vi "Apollo 3 v1.vi"() -> ()   [LabVIEW 2014]
uses:
  Global_vars.vi
panel:
  out "Test":dbl
  out "RL Command":dbl
  out "FR Command":dbl
  in  "Reorder Sim":i16=132
  out "Sim Lats and Longs":dbl[][](array[numeric]) format="%#_8g"
  in  "?":bool
  in  "Trail on/off":bool=TRUE
  in  "sim path":path=path "C:/Users/robotics/Desktop/Apollo II IGVC 2016 code/APOLLO 3 with fixed directory structure/Sim Drawings/IGVC II Test Paint.bmp"
  in  "Real WP Lats and Longs":dbl[][](array[numeric])=[[37.2651198, 81.2424197], [37.2652566, 81.2421218], [37.2653258, 81.2419709], [37.265326, 81.241971], [37.265326, 81.241971], [37.265326, 81.241971], [37.265326, 81.241971], [37.265326, 81.241971], [37.265326, 81.241971], [37.265326, 81.241971]] format="%#_8g"
  out "?":bool[](array[boolean])
  out "Robot Information":dbl[](array[numeric]) format="%#_8g"
  in  "Parameters":dbl[](array[numeric])=[2.0, 100.0, 10.0, 100.0, 30.0, 100.0, 3.0, 270.0, 37.1526, 81.2675, 7.3, 0.0, 60.0, 40.0, 0.0, 0.0, 0.0, 0.0, 0.0, 0.0]
  in  "GPS Port":refnum<visa-resource-name>="COM14"
  in  "Compass Port":refnum<visa-resource-name>="COM11"
  in  "Tx Prop  Port":refnum<visa-resource-name>="COM4"
  in  "Extra Port":refnum<visa-resource-name>="COM12"
  in  "Hokuyo Port":refnum<visa-resource-name>="COM13"
  out "main loop time":dbl=0.026001453399658203
  in  "Use ?\nOff       On":bool[](array[boolean])=[TRUE, TRUE, TRUE, TRUE, TRUE, FALSE]
  out "Local Map":picture
  in  "Num of WPs":i16=10
  out "Global Map":picture
  in  "START":bool
  in  "Mode:":bool
  out "WP Map":cluster{"WP Longs":dbl[], "WP Lats":dbl[]}(graph)
  out "loop iteration":i64=9025
  in  "STOP":bool
  # "Apollo 3 v1"
  # "Constants"
  # "Fat(0)"
  # "Setup"
  # "WT: Ahead(1)"
  # "WT: Gap(2)"
  # "WT: Slant(3)"
  # "GPS"
  # "WT: Dist(4)"
  # "LMS"
  # "WT: WP(5)"
  # "Vision"
  # "Sim Vel(6)"
  # "Tx Prop"
  # "Sim Hdg0(7)"
  # "Sim Lat0(8)"
  # "Comp"
  # "Sim Long0(9)"
  # "Extra"
  # "Sim Dev0(10)"
  # "Ang Bias(11)"
  # "Vel Bias(12)"
  # "Sim"
  # "Real"
  # "Run Time Robot Data"
  # "Goal x(13)"
  # "Goal y (14)"
  # "Robot Lat"
  # "Objx (15)"
  # "Robot Long"
  # "Objy (16)"
  # "Robot Heading"
  # "Old GPS L (17)"
  # "Robot Path Angle"
  # "Old GPS l (18)"
  # "Robot Speed"
  # "Simulation Settings"
  # "Old Heading (19)"
  # "Data Sent to Propeller"
  # "Angle to WP"
  # "Robot Trail:"
  # "Dist in Meters to WP"
  # "Pause"
  # "WP Number"
  # "Path to simulation BMP:"
  # "Next WP Lat"
  # "Resume"
  # "Next WP Long"
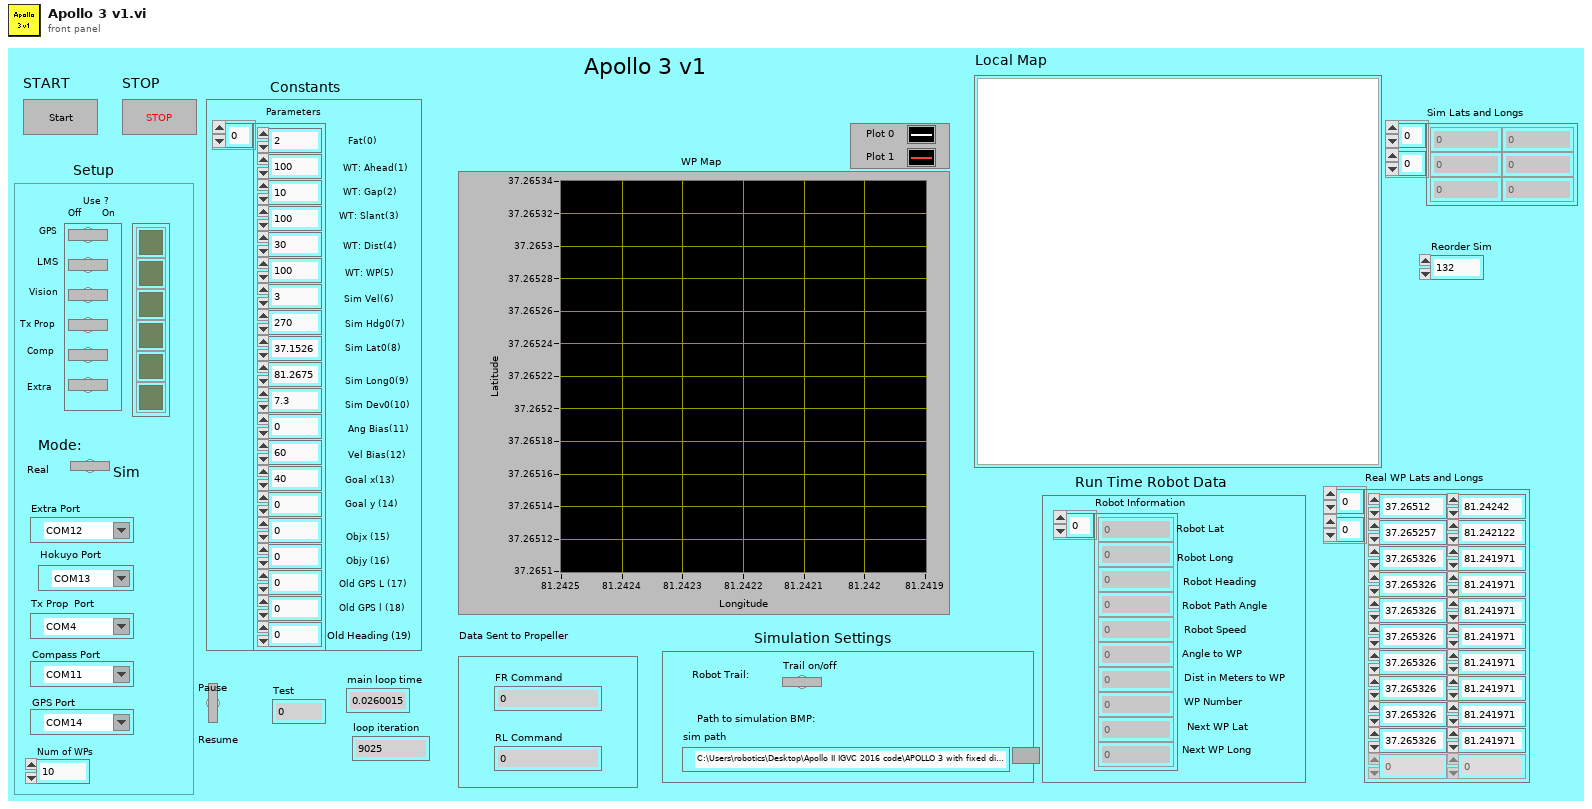
[diagram p1: front panel]
types:
  T1 = cluster{"     Use ?\nOff       On":bool[], "Mode:":bool, "Extra Port":refnum<visa-resource-name>, "Hokuyo Port":refnum<visa-resource-name>, "Tx Prop  Port":refnum<visa-resource-name>, "Compass Port":refnum<visa-resource-name>, "GPS Port":refnum<visa-resource-name>}
  T2 = cluster{"     Use ?\nOff       On":bool[], "Mode:":bool, "Extra Port":refnum<visa-resource-name>, "Hokuyo Port":refnum<visa-resource-name>, "Tx Prop  Port":refnum<visa-resource-name>, "Compass Port":refnum<visa-resource-name>, "GPS Port":refnum<visa-resource-name>, "Num of WPs":i16, "WP Lats and Longs":cluster{"WP Lats":dbl[], "WP Longs":dbl[]}, "Obst Lats and Longs":cluster{"Obst Lats":dbl[], "Obst Longs":dbl[]}, "Parameters":dbl[], "GPS Data":dbl[], "Compass":dbl, "LMS Vector":dbl[], "Vision Vector":dbl[], "Direction Cmd":dbl, "Speed Cmd":dbl, "WP Vector":dbl[], "WP Number":i32, "Extra":i16, "SW Map":i32[][], "Path Cluster":cluster{"Path x node":dbl[], "Path y node":dbl[]}, "Sim Course":i8[][]}
  T3 = cluster{"     Use ?\nOff       On":bool[], "Mode:":bool, "Extra Port":refnum<visa-resource-name>, "Hokuyo Port":refnum<visa-resource-name>, "Tx Prop Port":refnum<visa-resource-name>, "Compass Port":refnum<visa-resource-name>, "GPS Port":refnum<visa-resource-name>, "Num of WPs":i16, "WP Lats and Longs":cluster{"WP Lats":dbl[], "WP Longs":dbl[]}, "Obst Lats and Longs":cluster{"Obst Lats":dbl[], "Obst Longs":dbl[]}, "Parameters":dbl[], "GPS Data":dbl[], "Compass":dbl, "LMS Vector":dbl[], "Vision Vector":dbl[], "Direction Cmd":dbl, "Speed Cmd":dbl, "WP Vector":dbl[], "WP Number":i32, "Extra":i16, "SW Map":i32[][], "Path Cluster":cluster{"Path x node":dbl[], "Path y node":dbl[]}, "Sim Course":i8[][]}
  T4 = cluster{"     Use ?\nOff       On":bool[], "Mode:":bool, "Extra Port":refnum<visa-resource-name>, "Hokuyo Port":refnum<visa-resource-name>, "Prop  Port":refnum<visa-resource-name>, "Compass Port":refnum<visa-resource-name>, "GPS Port":refnum<visa-resource-name>, "Num of WPs":i16, "WP Lats and Longs":cluster{"WP Lats":dbl[], "WP Longs":dbl[]}, "Obst Lats and Longs":cluster{"Obst Lats":dbl[], "Obst Longs":dbl[]}, "Parameters":dbl[], "GPS Data":dbl[], "Compass":dbl, "LMS Vector":dbl[], "Vision Vector":dbl[], "Direction Cmd":dbl, "Speed Cmd":dbl, "WP Vector":dbl[], "WP Number":i32, "Extra":i16, "SW Map":i32[][], "Path Cluster":cluster{"Path x node":dbl[], "Path y node":dbl[]}, "Sim Course":i8[][]}
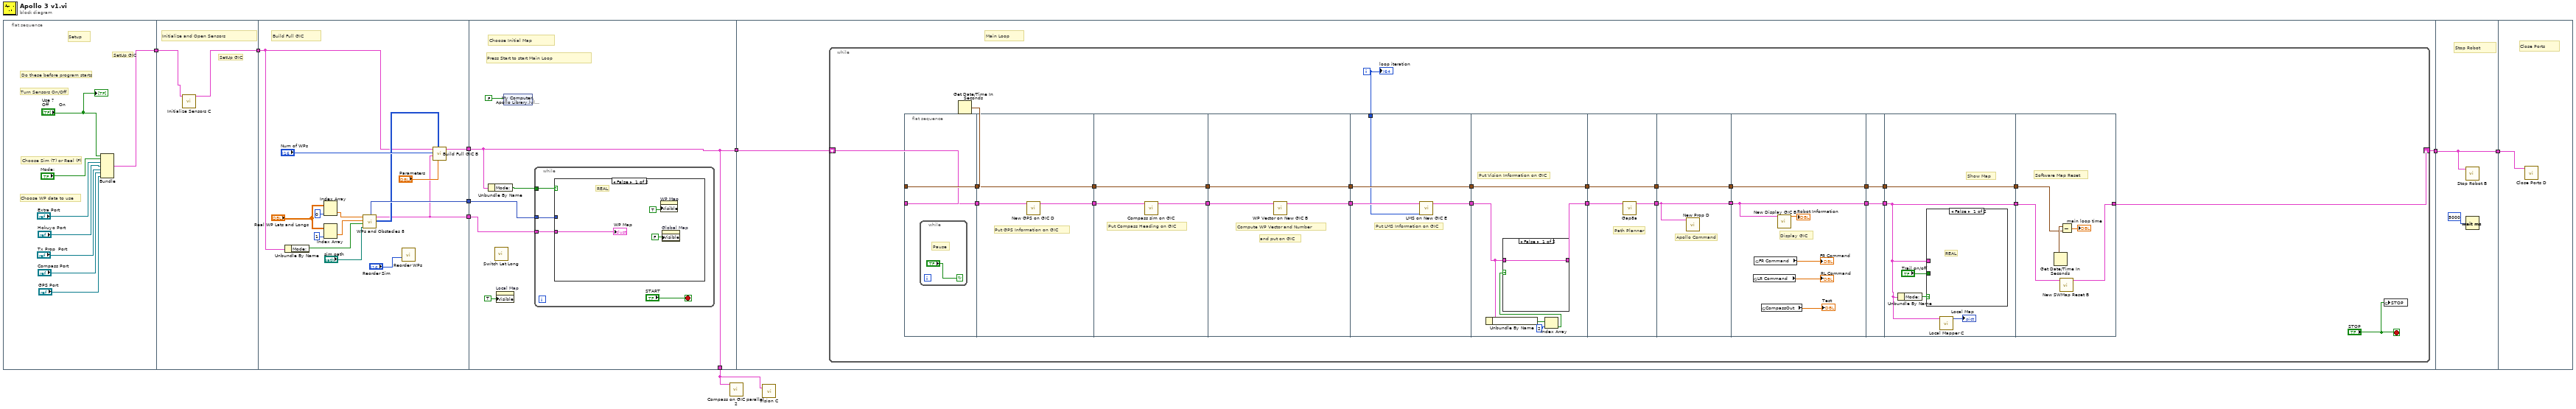
[diagram p0: block diagram]
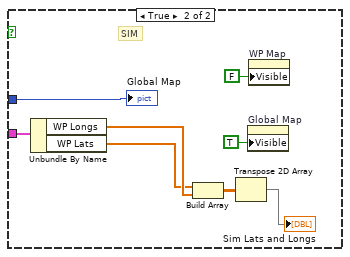
[diagram p2: hidden frame]
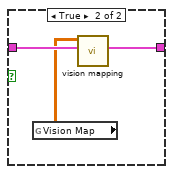
[diagram p3: hidden frame]
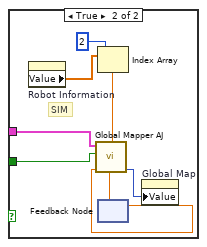
[diagram p4: hidden frame]
diagram:
  n1 = flat-sequence {
    tunnel: [w12] -> w9
    tunnel: w9 -> [w19]
    tunnel: [w18] -> w5
    tunnel: w5 -> [w24]
    tunnel: [w34] -> w4
    tunnel: [w32] -> w3
    tunnel: [w20] -> w2
    tunnel: [w35] -> w8
    tunnel: w2 -> [w36]
    tunnel: w3 -> [w38]
    tunnel: w4 -> [w35]
    tunnel: [w35] -> w1
    tunnel: [w57] -> w7
    tunnel: w8 -> [w56]
    tunnel: w7 -> [w143]
    tunnel: [w143] -> w6
    tunnel: w6 -> [w144]
    frame #0 {
      # "SetUp GIC"
      # "Choose WP data to use"
      # "Do these before program starts"
      # "Choose Sim (T) or Real (F)"
      # "Turn Sensors On/Off"
      # "Setup"
      n2 = Bundle("Use ?\nOff       On"="Use ?\nOff       On", "Mode:"="Mode:", "Extra Port"="Extra Port", "Hokuyo Port"="Hokuyo Port", "Tx Prop  Port"="Tx Prop  Port", "Compass Port"="Compass Port", "GPS Port"="GPS Port") -> (w12:T1)  [unwired: 1 in]
      "?" <- "Use ?\nOff       On"
    }
    frame #1 {
      # "SetUp GIC"
      # "Initialize and Open Sensors"
      n3 = call "Initialize Sensors C.vi"(11:w19) -> (3:w18:T1)  [unwired: 10 in]
    }
    frame #2 {
      # "Build Full GIC"
      n4 = Unbundle By Name(w24) -> ("Mode:"=w23:bool)
      n5 = Index Array(array="Real WP Lats and Longs", index (col)=1 ("disabled index (col)")) -> (element=w26:dbl[])  [unwired: 1 in]
      n6 = Index Array(array="Real WP Lats and Longs", index (col)=0 ("disabled index (col)")) -> (element=w27:dbl[])  [unwired: 1 in]
      n7 = call "WPs and Obstacles 8.vi"("sim path"="sim path", "Mode"=w23, "WP Real Longs"=w26, "WP Real Lats"=w27) -> ("Sim Matrx"=w31:u8[][], "WP Map"=w20:cluster{"WP Longs":dbl[], "WP Lats":dbl[]}, "Sim Course"=w32:picture)  [unwired: 3 in, 1 out]
      n8 = call "Reorder WPs.vi"("ReOrder Sim 123"="Reorder Sim") -> ()  [unwired: 10 in, 1 out]
      n9 = call "Build Full GIC B.vi"("Parameters"="Parameters", "Sim Course"=w31, "WP Lats and Longs"=w20, "Num of WPs"="Num of WPs", 11:w24) -> ("Full GIC"=w34:T2)  [unwired: 6 in]
    }
    frame #3 {
      # "Choose Initial Map"
      # "Press Start to start Main Loop"
      n10 = Unbundle By Name(w35) -> ("Mode:"=w37:bool)
      n11 = call "Switch Lat Long.vi"() -> ()  [unwired: 1 in, 1 out]
      n12 = property on="Local Map" class="Pict"("Visible"=TRUE) -> ()  [unwired: 2 in, 2 out]
      n13 = shared-variable "My Computer\\Apollo Library.lvlib\\stop"(FALSE) -> ()  [unwired: 1 in, 1 out]
      n14 = while {
        tunnel: w38 -> [w42]
        tunnel: w36 -> [w41]
        tunnel: w37 -> [w43]
        stop <- "START" stop-if-true
        n15 = case shown="False" w43 {
          tunnel: w42 -> [_ w55]
          tunnel: w41 -> [w47 w52]
          frame False {
            # "REAL"
            n16 = property on="WP Map" class="XYGraph (strict)"("Visible"=TRUE) -> ()  [unwired: 2 in, 2 out]
            n17 = property on="Global Map" class="Pict"("Visible"=FALSE) -> ()  [unwired: 2 in, 2 out]
            "WP Map" <- w47
          }
          frame True {
            # "SIM"
            n18 = Unbundle By Name(w52) -> ("WP Longs"=w51:dbl[], "WP Lats"=w50:dbl[])
            n19 = Build Array(w50, w51) -> (w49:dbl[][])
            n20 = Transpose 2D Array(2D array=w49) -> (transposed array=→"Sim Lats and Longs":dbl[][])
            n21 = property on="Global Map" class="Pict"("Visible"=TRUE) -> ()  [unwired: 2 in, 2 out]
            n22 = property on="WP Map" class="XYGraph (strict)"("Visible"=FALSE) -> ()  [unwired: 2 in, 2 out]
            "Global Map" <- w55
          }
        }
      }
    }
    frame #4 {
      # "Main Loop"
      n23 = while {
        shift-right: [w67] -> w57
        shift-left: w56 -> [w75]
        i -> [w66]
        stop <- "STOP" stop-if-true
        n24 = flat-sequence {
          tunnel: w75 -> [w85]
          tunnel: w78 -> [w86]
          tunnel: [w86] -> w61
          tunnel: [w85] -> w60
          tunnel: [w90] -> w79
          tunnel: [w88] -> w74
          tunnel: w61 -> [w90]
          tunnel: w60 -> [w89]
          tunnel: [w93] -> w80
          tunnel: w79 -> [w93]
          tunnel: w74 -> [w92]
          tunnel: [w91] -> w73
          tunnel: [w96] -> w81
          tunnel: w80 -> [w96]
          tunnel: w73 -> [w95]
          tunnel: [w94] -> w72
          tunnel: [w100] -> w82
          tunnel: w81 -> [w100]
          tunnel: w72 -> [w99]
          tunnel: [w98] -> w71
          tunnel: w66 -> [w97]
          tunnel: [w106] -> w77
          tunnel: w82 -> [w106]
          tunnel: w71 -> [w102]
          tunnel: [w101] -> w59
          tunnel: [w113] -> w76
          tunnel: w77 -> [w113]
          tunnel: [w111] -> w70
          tunnel: w59 -> [w112]
          tunnel: [w115] -> w83
          tunnel: w76 -> [w115]
          tunnel: w70 -> [w114]
          tunnel: [w114] -> w69
          tunnel: [w121] -> w65
          tunnel: w83 -> [w121]
          tunnel: w69 -> [w119]
          tunnel: [w119] -> w63
          tunnel: w65 -> [w123]
          tunnel: [w123] -> w64
          tunnel: w63 -> [w122]
          tunnel: [w122] -> w62
          tunnel: [w128] -> w84
          tunnel: w64 -> [w128]
          tunnel: w62 -> [w124]
          tunnel: [w124] -> w68
          tunnel: w84 -> [w139]
          tunnel: w68 -> [w138]
          tunnel: [w137] -> w67
          frame #0 {
            n25 = while {
              stop <- "?" continue-if-true
              # "Pause"
            }
          }
          frame #1 {
            # "Put GPS Information on GIC"
            n26 = call "New GPS on GIC D.vi"("GIC Input"=w89) -> ("GIC Output"=w88:T2)  [unwired: 10 in]
          }
          frame #2 {
            # "Put Compass Heading on GIC"
            n27 = call "Compass sim on GIC.vi"("GIC Input"=w92) -> ("GIC Output"=w91:T2)  [unwired: 10 in]
          }
          frame #3 {
            # "and put on GIC"
            # "Compute WP Vector and Number"
            n28 = call "WP Vector on New GIC B.vi"("GIC Input"=w95) -> ("GIC Output"=w94:T2)  [unwired: 10 in]
          }
          frame #4 {
            # "Put LMS Information on GIC"
            n29 = call "LMS on New GIC E.vi"("Iteration num"=w97, "GIC Input"=w99) -> ("GIC Output"=w98:T2)  [unwired: 9 in]
          }
          frame #5 {
            # "Put Vision Information on GIC"
            n30 = Unbundle By Name(w102) -> ("Use ?\nOff       On"=w105:bool[])
            n31 = Index Array(array=w105, index=2) -> (element=w103:bool)
            n32 = case shown="False" w103 {
              tunnel: w102 -> [w107 w110]
              tunnel: [w107 w109] -> w101
              frame False {
              }
              frame True {
                n33 = global read "Global_vars.vi" "Vision Map"() -> (w108:dbl[][])
                n34 = call "vision mapping.vi"("GIC Input"=w110, "From vision processing"=w108) -> ("GIC Output"=w109:T3)  [unwired: 9 in]
              }
            }
          }
          frame #6 {
            # "Path Planner"
            n35 = call "Gap8a.vi"("GIC Input"=w112) -> ("GIC Output"=w111:T3)  [unwired: 10 in]
          }
          frame #7 {
            # "Apollo Command"
            n36 = call "New Prop D.vi"("GIC Input"=w114) -> ()  [unwired: 11 in]
          }
          frame #8 {
            # "Display GIC"
            n37 = global read "Global_vars.vi" "LR Command"() -> (→"RL Command":dbl)
            n38 = global read "Global_vars.vi" "FR Command"() -> (→"FR Command":dbl)
            n39 = global read "Global_vars.vi" "CompassOut"() -> (→"Test":dbl)
            n40 = call "New Display GIC B.vi"("GIC Input"=w119) -> ("Array"=→"Robot Information":dbl[])  [unwired: 10 in]
          }
          frame #9 {
          }
          frame #10 {
            # "Show Map"
            n41 = Unbundle By Name(w124) -> ("Mode:"=w127:bool)
            n42 = case shown="False" w127 {
              tunnel: "Trail on/off" -> [_ w135]
              tunnel: w124 -> [_ w134]
              frame False {
                # "REAL"
              }
              frame True {
                # "SIM"
                n43 = property on="Robot Information" class="Arr (strict)"() -> ("Value"=w132:dbl[])  [unwired: 2 in, 2 out]
                n44 = Index Array(array=w132, index=2) -> (element=w131:dbl)
                n45 = feedback #1() -> (w129:dbl)  [unwired: 1 in]
                n46 = call "Global Mapper AJ.vi"("Old Heading"=w129, "Heading"=w131, "Trail off/on"=w135, "GIC Input"=w134) -> ("picture out"=w136:picture, "Old Heading Out"=w130:dbl)  [unwired: 6 in]
                n47 = feedback-in #1(w130) -> ()
                n48 = property on="Global Map" class="Pict"("Value"=w136) -> ()  [unwired: 2 in, 2 out]
              }
            }
            n49 = call "Local Mapper C.vi"("GIC Input"=w124) -> ("Local Map"=→"Local Map":picture)  [unwired: 10 in]
          }
          frame #11 {
            # "Software Map Reset"
            n50 = Get Date/Time In Seconds() -> (seconds since 1Jan1904=w140:timestamp)
            n51 = call "New SWMap Reset B.vi"("GIC Input"=w138) -> ("GIC Output"=w137:T4)  [unwired: 10 in]
            n52 = Subtract(x=w140, y=w139) -> (x-y=→"main loop time":dbl)
          }
        }
        n53 = Get Date/Time In Seconds() -> (seconds since 1Jan1904=w78:timestamp)
        n54 = global write "Global_vars.vi" "STOP"("STOP") -> ()
        "loop iteration" <- w66
      }
    }
    frame #5 {
      # "Stop Robot"
      n55 = call "Stop Robot B.vi"("GIC Input"=w143) -> ()  [unwired: 11 in]
      n56 = Wait (ms)(milliseconds to wait=5000) -> ()  [unwired: 1 out]
    }
    frame #6 {
      # "Close Ports"
      n57 = call "Close Ports D.vi"("GIC Input"=w144) -> ()  [unwired: 11 in]
    }
  }
  n58 = call "Compass on GIC parallel 2.vi"("GIC Input 2"=w1) -> ()  [unwired: 11 in]
  n59 = call "vision C.vi"("GIC Input"=w1) -> ()  [unwired: 2 in, 1 out]
